vi "Filter (G3)-Compute Scale Factor.vi"(0 "Filter":T1={"Type"=enum."Lowpass", "CF (kHz)"=0.0, "BW (kHz)"=0.0, "Cascade"=FALSE, "Quadrature"=FALSE, "Scale Factor"=0.0, "Stages"=[], "Class"=enum."Elliptic", "Order"=0, "BWUnits"=enum."Linear"} {"Stages"."IIR Filter"."Forward Coefficients" format="%.4f"; "Stages"."IIR Filter"."Reverse Coefficients" format="%.4f"}, 7 "Sampling Rate (Hz)":dbl, 11 "error in (no error)":errorcluster) -> (4 "Filter out":T1={"Type"=enum."Lowpass", "CF (kHz)"=0.0, "BW (kHz)"=0.0, "Cascade"=FALSE, "Quadrature"=FALSE, "Scale Factor"=0.0, "Stages"=[], "Class"=enum."Elliptic", "Order"=0, "BWUnits"=enum."Linear"} {"Stages"."IIR Filter"."Forward Coefficients" format="%.4f"; "Stages"."IIR Filter"."Reverse Coefficients" format="%.4f"}, 15 "error out":errorcluster)   [LabVIEW 2020]
uses:
  XControls/Filter (G3)/Filter Data.ctl
  XControls/Filter (G3)/Filter Type.ctl
  Filter VIs/Filter-Bandwidth Units.ctl
  <vilib>/Analysis/1siggen.llb/Ramp Pattern by Samples.vi
  <vilib>/Analysis/5stat.llb/RMS (DBL).vi
  <vilib>/Analysis/NI_AALBase.lvlib
  <vilib>/Analysis/NI_AALPro.lvlib
  XControls/Filter (G3)/Filter (G3).xctl
panel:
  out "RMS":dbl
  out "Scale Factor":dbl
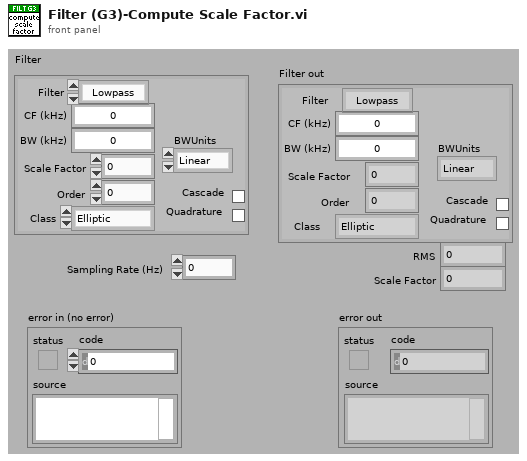
[diagram p1: front panel]
types:
  T1 = typedef "Filter (G3).xctl/Filter Data.ctl" = cluster{"Type":T2, "CF (kHz)":dbl, "BW (kHz)":dbl, "Cascade":bool, "Quadrature":bool, "Scale Factor":dbl, "Stages":cluster{"IIR Filter":cluster{"filter structure":enum32{"IIR 2nd Order", "IIR 4th Order"}, "Reverse Coefficients":dbl[], "Forward Coefficients":dbl[]}, "State":dbl[]}[], "Class":enum16{"Elliptic", "Butterworth"}, "Order":i32, "BWUnits":T3}
  T2 = typedef "Filter (G3).xctl/Filter Type.ctl" = enum16{"OFF", "Lowpass", "Highpass", "Bandpass", "Bandstop"}
  T3 = typedef "Filter-Bandwidth Units.ctl" = enum16{"Linear", "Octaves", "Min-Max"}
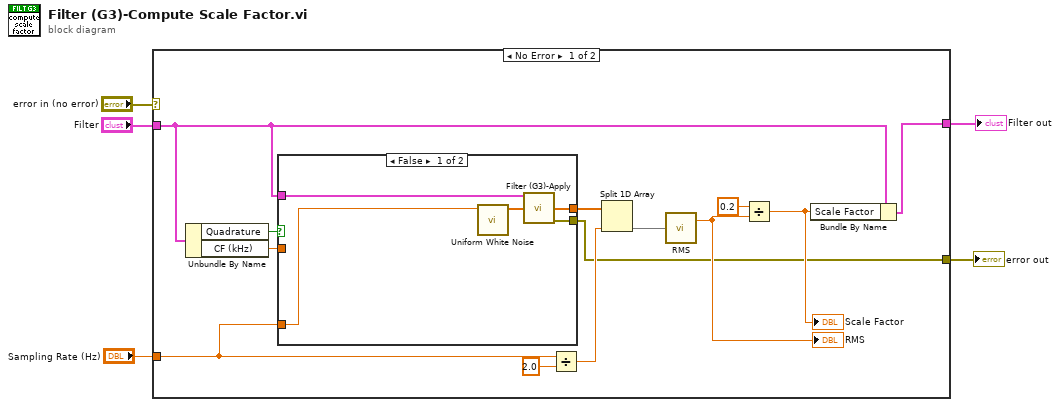
[diagram p0: block diagram]
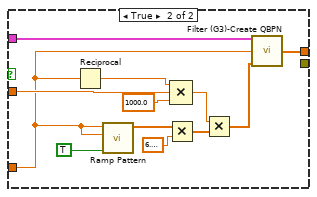
[diagram p2: hidden frame]
diagram:
  n1 = case shown="No Error" "error in (no error)" {
    selector: "error in (no error)" -> [_ w37]
    tunnel: "Filter" -> [w9 w36]
    tunnel: [w18 w36] -> w4
    tunnel: [w6 w37] -> w2
    tunnel: "Sampling Rate (Hz)" -> [w14 _]
    frame No Error {
      n2 = Unbundle By Name(w9) -> ("Quadrature"=w8:bool, "CF (kHz)"=w7:dbl)
      n3 = case shown="False" w8 {
        tunnel: w9 -> [w23 w34]
        tunnel: [w21 w35] -> w15
        tunnel: w14 -> [w20 w25]
        tunnel: w7 -> [_ w26]
        tunnel: [w19 _] -> w6
        frame False {
          n4 = call <vilib>:"Uniform White Noise.vi"("samples"=w20) -> ("uniform white noise"=w22:dbl[])  [unwired: 9 in, 1 out]
          n5 = call "Filter (G3)-Apply.vi"("Filter"=w23, "X"=w22) -> ("Filtered X"=w21:dbl[], "error out"=w19:errorcluster)  [unwired: 11 in, 1 out]
        }
        frame True {
          n6 = Reciprocal(x=w25) -> (1/x=w33:dbl)
          n7 = call-poly <vilib>:"Ramp Pattern.vi"("exclude end?"=TRUE, "end"=w25, "samples"=w25) -> ("Ramp Pattern"=w28:dbl[])  [unwired: 7 in, 1 out]
          n8 = Multiply(x=w28, y=6.283185307179586) -> (x*y=w29:dbl[])
          n9 = Compound Arithmetic op=MULTIPLY(w33, w26, 1000.0 ("y")) -> (w31:dbl)
          n10 = Multiply(x=w31, y=w29) -> (x*y=w24:dbl[])
          n11 = call "Filter (G3)-Create QBPN.vi"("Filter"=w34, "Npts"=w25, "Omega (t)"=w24) -> ("BP noise"=w35:dbl[])  [unwired: 11 in, 1 out]
        }
      }
      n12 = Divide(x=w14, y=2.0) -> (x/y=w12:dbl)
      n13 = Split 1D Array(array=w15, index=w12) -> (second subarray=w11:dbl[])  [unwired: 1 out]
      n14 = call-poly <vilib>:"RMS.vi"("X"=w11) -> ("rms value"=w10:dbl)  [unwired: 1 out]
      "RMS" <- w10
      n15 = Divide(x=0.2, y=w10) -> (x/y=w16:dbl)
      "Scale Factor" <- w16
      n16 = Bundle By Name(cluster=w9, "Scale Factor"=w16) -> (w18:T1)
    }
    frame Error {
    }
  }
  "error out" <- w2
  "Filter out" <- w4
